vi "RT_AInoiseMeas.vi"() -> ()   [LabVIEW 2020]
uses:
  <vilib>/NI/STM/SubVIs/MetaDataElement.ctl
  <vilib>/Platform/TimedLoop/XDataNode/timing_clust.ctl
  <vilib>/Platform/TimedLoop/XDataNode/nitl_modes.ctl
  <vilib>/Platform/TimedLoop/XDataNode/wakeup.ctl
  <vilib>/NI/STM/TCP/Write Meta Data (TCP Ref).vi
  <vilib>/NI/STM/TCP/Get Connection Reference (TCP).vi
  <vilib>/NI/STM/TCP/Write Meta Data (TCP Clst).vi
  <vilib>/FPGAPlugInAG/cRIO-9064/niLvFpga_Open_cRIO-9064.vi
  <vilib>/rvi/interface/common/dynamic/niFpgaDynamicAddResources.vi
  <vilib>/NI/STM/TCP/Write Message (TCP).vi
  <vilib>/Utility/error.llb/Error Cluster From Error Code.vi
  <vilib>/rvi/errors/niLvFpgaAdjustHostInterfaceError.vi
  <vilib>/FPGAPlugInAG/Dynamic/niLvFpga_Close_Dynamic.vi
  <vilib>/rvi/interface/nirviOpenFPGA/nirviOpenFPGA.xnode
  FPGA Bitfiles/pumpmeasurements_FPGATarget2_FPGAmain_llEPu4umcUg.lvbitx
  <vilib>/rvi/interface/nirviReadWriteControl/nirviReadWriteControl.xnode
  <vilib>/Platform/TimedLoop/XDataNode/XDataNode.xnode
  <vilib>/rvi/interface/nirviCloseFPGA/nirviCloseFPGA.xnode
  <vilib>/Platform/TimedLoop/XDataNode/XDNodeRunTimeDep.lvlib
  Components_global/Timing/Timing.lvlib
  <vilib>/NI/STM/NI STM.lvlib
  <vilib>/rvi/interface/Simulation/niFpgaSimulationCallBeginRW.vi
  NiFpgaLv.dll
panel:
  out "NI9208 AI \nloop time [ms]":u32
  out "NI9205 AI \nloop time [ms]":dbl
  in  "Select channel":T1(ring)
  in  "Select Module":enum16{"NI9205", "NI9208"}(ring)
  out "RT Loop Rate":dbl format="%.3p"
  out "# of iterations\n[STM write]":i32
  out "# elements \nFIFO buffer":u32
  out "Finished \nlate counter?":dbl
  in  "stop":bool
  # "- Open PC_AINoiseMeas.vi and run that VI \nas well to start capturing data!"
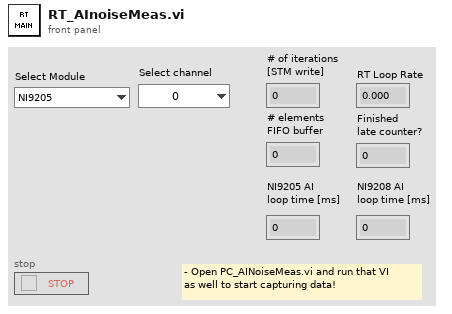
[diagram p1: front panel]
types:
  T1 = enum16{"0", "1", "2", "3", "4", "5", "6", "7", "8", "9", "10", "11", "12", "13", "14", "15"}
  T2 = typedef "NI STM.lvlib/MetaDataElement.ctl" = string
  T3 = typedef "NI STM.lvlib/TCP Connection Info.ctl" = cluster{"connection ID":refnum<k5>, "meta data":T2[]}
  T4 = typedef "XDNodeRunTimeDep.lvlib/timing_clust.ctl" = cluster{"Expected End [f-1]":u64, "Actual End [f-1]":u64, "Finished Late? [f-1]":bool, "Expected End [i-1]":u64, "Actual End [i-1]":u64, "Finished Late? [i-1]":bool, "Expected Start [i]":u64, "Actual Start [i]":u64, "Expected Start [f]":u64, "Actual Start [f]":u64, "Source Name":string, "Structure Name":string, "Period":i64, "Deadline":i64, "Offset":i64, "Start":i64, "Priority":i32, "Timeout":i32, "Mode":T5, "Wakeup Reason":T6, "Error":errorcluster, "Source Type":string, "Secondary Source Type":string, "Global End Time":u64, "Global Start Time":u64, "Frame Duration":u64, "Iteration Duration":u64, "Assigned CPU":i32, "I/O Scan Engine Mode":u32}
  T5 = typedef "XDNodeRunTimeDep.lvlib/nitl_modes.ctl" = enum32{"No Change", "Process missed periods, maintain original phase", "Discard missed periods, maintain original phase", "Process missed periods, ignore original phase", "Discard missed periods, ignore original phase"}
  T6 = typedef "XDNodeRunTimeDep.lvlib/wakeup.ctl" = enum32{"Normal", "Aborted", "Asynchronous wakeup", "Timing source error", "Timed loop error", "Timeout"}
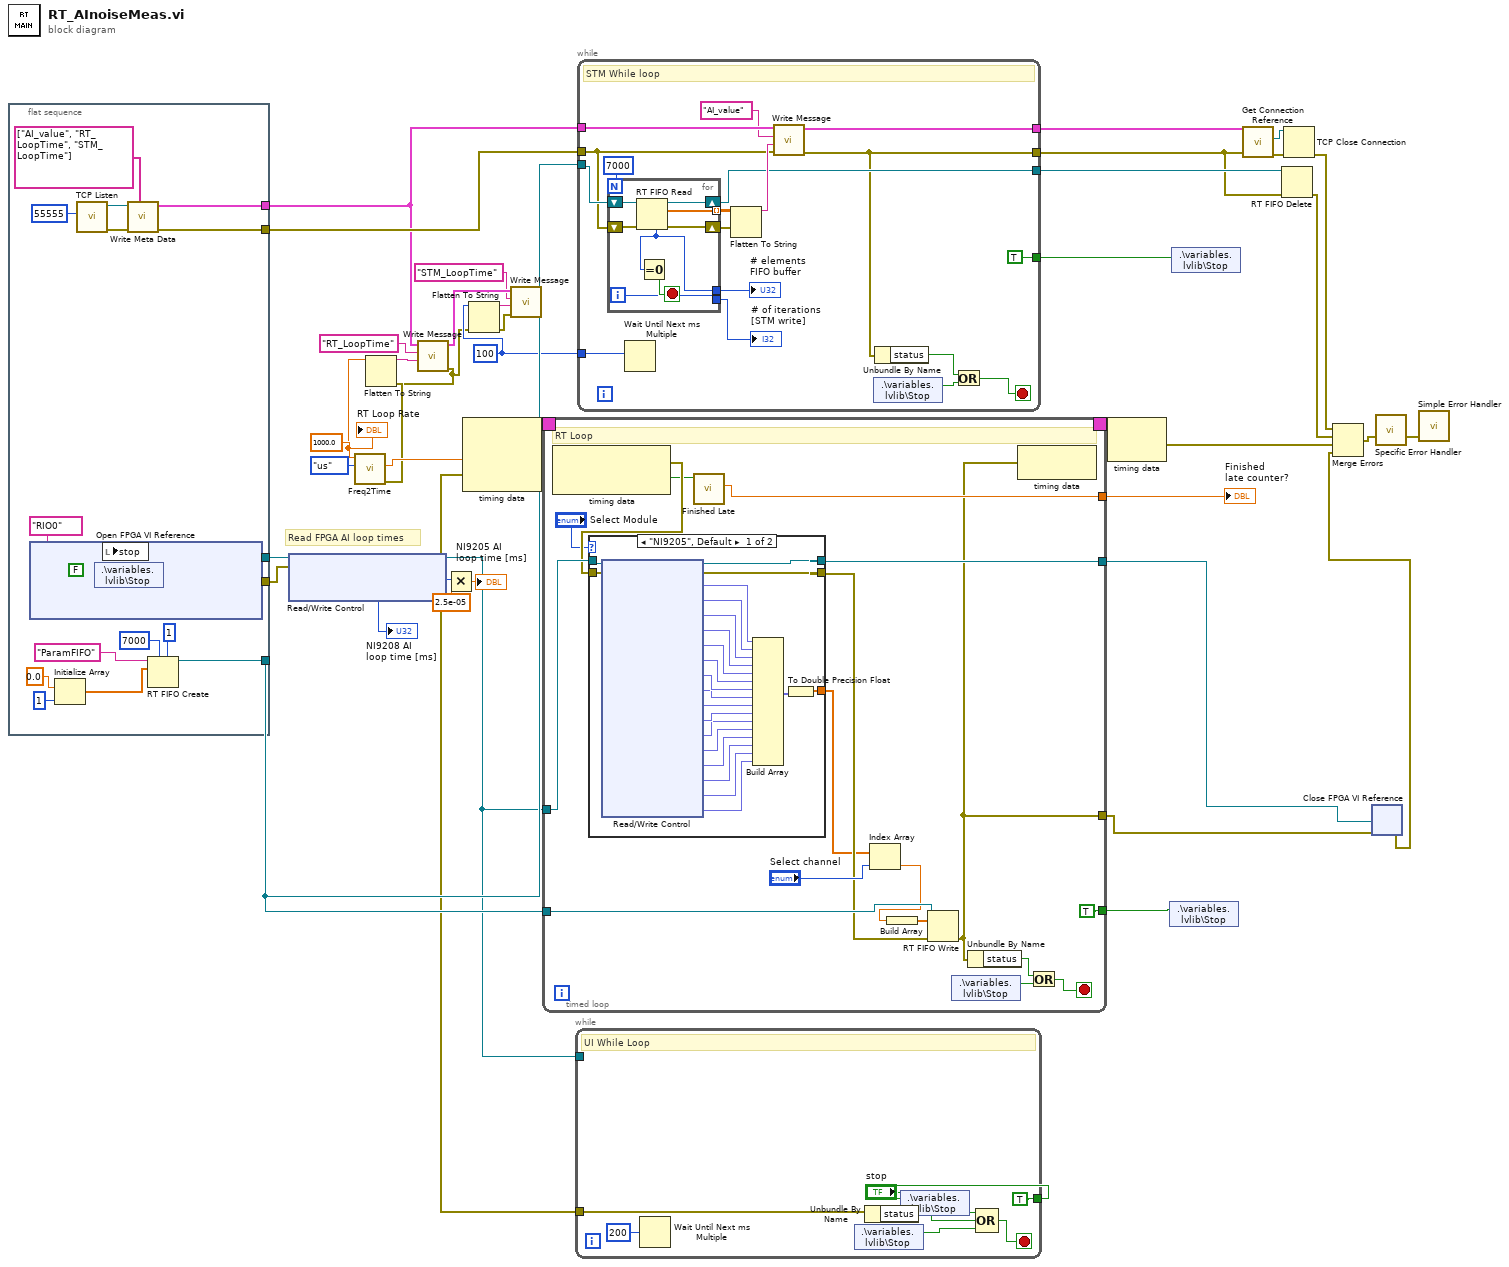
[diagram p0: block diagram]
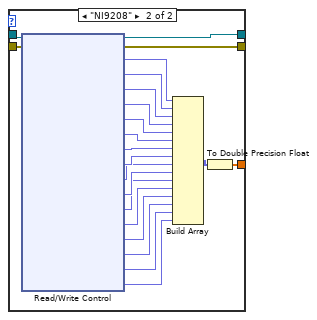
[diagram p2: hidden frame]
diagram:
  w17 = u32 100 ("millisecond multiple")
  # "Read FPGA AI loop times"
  n1 = flat-sequence {
    tunnel: [w59] -> w8
    tunnel: [w58] -> w1
    tunnel: [w53] -> w14
    tunnel: [w52] -> w37
    tunnel: [w51] -> w18
    frame #0 {
      w60 = FALSE ("Stop")
      n2 = xnode "Open FPGA VI Reference"("resource name"=tag "RIO0") -> ("FPGA VI Reference Out"=w58:refnum<k20>, "error out"=w61:errorcluster)  [unwired: 1 in]
      n3 = Initialize Array(0.0 ("element"), 1 ("dimension size")) -> (w46:dbl[])
      n4 = call <vilib>:"TCP Listen.vi"("port"=u16 55555) -> ("error out"=w56:errorcluster, "connection ID"=w55:refnum<k5>)  [unwired: 6 in, 3 out]
      n5 = shared-variable ".\\variables.lvlib\\Stop"(w60, error in=w61) -> (error out=w59:errorcluster)
      n6 = local write "stop"(w60) -> ()
      n7 = call-poly <vilib>:"Write Meta Data.vi"("meta data"=T2[] ["AI_value", "RT_LoopTime", "STM_LoopTime"], "error in"=w56, "connection ID"=w55) -> ("error out"=w52:errorcluster, "connection info out"=w53:T3)  [unwired: 7 in]
      n8 = RT FIFO Create(0:"ParamFIFO" ("name (unnamed)"), 1:w46, 4:u32 7000 ("size (10)"), 6:u32 1 ("elements in array (1)")) -> (8:w51:refnum<k33>)  [unwired: 4 in, 2 out]
    }
  }
  n9 = xnode "Read/Write Control"("FPGA VI Reference In"=w1, "error in"=w8) -> ("FPGA VI Reference Out"=w6:refnum<k20>, "error out"=w7:errorcluster, "NI9205 AI loop time [ticks]"=w2:u32, "NI9208 AI loop time [ms]"=→"NI9208 AI \nloop time [ms]":u32)
  n10 = call "Freq2Time.vi"("Int. Time Unit"=enum16{"sec", "us", "ms"}."us", "Sample rate (Hz)"=1000.0 ("Period")) -> ("error out"=w26:errorcluster, "Int.  time [unit]"=w38:dbl, "New Sample rate (Hz)"=w28:dbl)  [unwired: 7 in]
  "RT Loop Rate" <- w28
  n11 = Flatten To String(anything=w28, error in (no error)=w26) -> (data string=w29:string, error out=w16:errorcluster)  [unwired: 2 in, 1 out]
  n12 = call-poly <vilib>:"Write Message.vi"("error in"=w16, "data"=w29, "name"="RT_LoopTime", "connection info in"=w14) -> ("connection info out"=w13:T3)  [unwired: 6 in, 1 out]
  n13 = Multiply(x=w2, y=2.5e-05 ("NI9205 AI loop time [ms]")) -> (x*y=→"NI9205 AI \nloop time [ms]":dbl)
  n14 = node-c288(w38, w7) -> (w43:T4)  [unwired: 1 in]
  n15 = Flatten To String(anything=w17, error in (no error)=w16) -> (data string=w11:string, error out=w15:errorcluster)  [unwired: 2 in, 1 out]
  n16 = call-poly <vilib>:"Write Message.vi"("error in"=w15, "data"=w11, "name"="STM_LoopTime", "connection info in"=w13) -> ()  [unwired: 6 in, 2 out]
  n17 = timed-loop {
    tunnel: w6 -> [w78]
    timing: w43 -> [_]
    timing-out: [_] -> w42
    tunnel: [w75] -> w41
    tunnel: w18 -> [w74]
    tunnel: [TRUE ("Stop")] -> w20
    tunnel: [w66] -> w10
    tunnel: [w65] -> w9
    stop <- w72 stop-if-true
    # "RT Loop"
    n18 = node-c288() -> (w77:errorcluster, w76:bool)  [unwired: 1 in]
    n19 = case shown="\"NI9205\", Default" "Select Module" {
      tunnel: w78 -> [w100 w122]
      tunnel: w77 -> [w99 w120]
      tunnel: [w79 w103] -> w63
      tunnel: [w98 w121] -> w66
      tunnel: [w97 w119] -> w68
      frame "NI9205", Default {
        n20 = xnode "Read/Write Control"("FPGA VI Reference In"=w100, "error in"=w99) -> ("FPGA VI Reference Out"=w98:refnum<k20>, "error out"=w97:errorcluster, "NI9205: AI0 [V]"=w96:fxp<+/-,35,5>, "NI9205: AI1 [V]"=w95:fxp<+/-,35,5>, "NI9205: AI2 [V]"=w94:fxp<+/-,35,5>, "NI9205: AI3 [V]"=w93:fxp<+/-,35,5>, "NI9205: AI4 [V]"=w92:fxp<+/-,35,5>, "NI9205: AI5 [V]"=w91:fxp<+/-,35,5>, "NI9205: AI6 [V]"=w90:fxp<+/-,35,5>, "NI9205: AI7 [V]"=w89:fxp<+/-,35,5>, "NI9205: AI16 [V]"=w88:fxp<+/-,35,5>, "NI9205: AI17 [V]"=w87:fxp<+/-,35,5>, "NI9205: AI18 [V]"=w86:fxp<+/-,35,5>, "NI9205: AI19 [V]"=w85:fxp<+/-,35,5>, "NI9205: AI20 [V]"=w84:fxp<+/-,35,5>, "NI9205: AI21 [V]"=w83:fxp<+/-,35,5>, "NI9205: AI22 [V]"=w82:fxp<+/-,35,5>, "NI9205: AI23 [V]"=w81:fxp<+/-,35,5>)
        n21 = Build Array(w96, w95, w94, w93, w92, w91, w90, w89, w88, w87, w86, w85, w84, w83, w82, w81) -> (w80:fxp<+/-,35,5>[])
        n22 = To Double Precision Float(number=w80) -> (double precision float=w79:dbl[])
      }
      frame "NI9208" {
        n23 = xnode "Read/Write Control"("FPGA VI Reference In"=w122, "error in"=w120) -> ("FPGA VI Reference Out"=w121:refnum<k20>, "error out"=w119:errorcluster, "NI9208: AI0 [A]"=w101:fxp<+/-,24,-4>, "NI9208: AI1 [A]"=w118:fxp<+/-,24,-4>, "NI9208: AI2 [A]"=w117:fxp<+/-,24,-4>, "NI9208: AI3 [A]"=w116:fxp<+/-,24,-4>, "NI9208: AI4 [A]"=w115:fxp<+/-,24,-4>, "NI9208: AI5 [A]"=w114:fxp<+/-,24,-4>, "NI9208: AI6 [A]"=w113:fxp<+/-,24,-4>, "NI9208: AI7 [A]"=w112:fxp<+/-,24,-4>, "NI9208: AI8 [A]"=w111:fxp<+/-,24,-4>, "NI9208: AI9 [A]"=w110:fxp<+/-,24,-4>, "NI9208: AI10 [A]"=w109:fxp<+/-,24,-4>, "NI9208: AI11 [A]"=w108:fxp<+/-,24,-4>, "NI9208: AI12 [A]"=w107:fxp<+/-,24,-4>, "NI9208: AI13 [A]"=w106:fxp<+/-,24,-4>, "NI9208: AI14 [A]"=w105:fxp<+/-,24,-4>, "NI9208: AI15 [A]"=w104:fxp<+/-,24,-4>)
        n24 = Build Array(w101, w118, w117, w116, w115, w114, w113, w112, w111, w110, w109, w108, w107, w106, w105, w104) -> (w102:fxp<+/-,24,-4>[])
        n25 = To Double Precision Float(number=w102) -> (double precision float=w103:dbl[])
      }
    }
    n26 = call "Finished Late.vi"("Finished \nLate?"=w76) -> ("# Finished\nLate counter"=w75:dbl)  [unwired: 8 in, 2 out]
    n27 = Index Array(array=w63, index="Select channel") -> (element=w64:dbl)
    n28 = Build Array(w64) -> (w62:dbl[])
    n29 = RT FIFO Write(0:w74, 1:w62, 3:w68) -> (11:w65:errorcluster)  [unwired: 2 in, 3 out]
    n30 = shared-variable ".\\variables.lvlib\\Stop"() -> (w71:bool)  [unwired: 1 in, 1 out]
    n31 = Unbundle By Name(w65) -> ("status"=w70:bool)
    n32 = node-c288(w65) -> ()  [unwired: 1 out]
    n33 = Or(x=w70, y=w71) -> (x .or. y?=w72:bool)
  }
  "Finished \nlate counter?" <- w41
  n34 = while {
    tunnel: w7 -> [w131]
    tunnel: w6 -> [_]
    tunnel: [TRUE ("Stop")] -> w19
    stop <- w132 stop-if-true
    # "UI While Loop"
    n35 = Wait Until Next ms Multiple(millisecond multiple=u32 200) -> ()  [unwired: 1 out]
    n36 = shared-variable ".\\variables.lvlib\\Stop"() -> (w133:bool)  [unwired: 1 in, 1 out]
    n37 = Unbundle By Name(w131) -> ("status"=w130:bool)
    n38 = Compound Arithmetic op=OR("stop", w130, w133) -> (w132:bool)
  }
  n39 = while {
    tunnel: w14 -> [w153]
    tunnel: w37 -> [w147]
    tunnel: [w151] -> w36
    tunnel: [w137] -> w32
    tunnel: w18 -> [w149]
    tunnel: [w146] -> w33
    tunnel: [TRUE ("Stop")] -> w21
    tunnel: w17 -> [w136]
    stop <- w139 stop-if-true
    # "STM While loop"
    n40 = for {
      N: 7000 -> [_]
      shift-right: [w158] -> w146
      shift-left: w149 -> [w161]
      shift-right: [w160] -> w148
      shift-left: w147 -> [w159]
      tunnel: [w157] -> w145
      tunnel: [w155] -> w144
      tunnel: [w154] -> w143 mode=indexing
      i -> [w155]
      stop <- w156 stop-if-true
      n41 = RT FIFO Read(0:w161, 3:w159) -> (7:w157:u32, 8:w158:refnum<k33>, 9:w154:dbl[], 11:w160:errorcluster)  [unwired: 2 in, 1 out]
      n42 = Equal To 0?(x=w157) -> (x = 0?=w156:bool)
    }
    "# elements \nFIFO buffer" <- w145
    "# of iterations\n[STM write]" <- w144
    n43 = Wait Until Next ms Multiple(millisecond multiple=w136) -> ()  [unwired: 1 out]
    n44 = Flatten To String(anything=w143, error in (no error)=w148) -> (data string=w150:string)  [unwired: 2 in, 2 out]
    n45 = call-poly <vilib>:"Write Message.vi"("error in"=w147, "data"=w150, "name"="AI_value", "connection info in"=w153) -> ("error out"=w137:errorcluster, "connection info out"=w151:T3)  [unwired: 6 in]
    n46 = shared-variable ".\\variables.lvlib\\Stop"() -> (w140:bool)  [unwired: 1 in, 1 out]
    n47 = Unbundle By Name(w137) -> ("status"=w138:bool)
    n48 = Or(x=w138, y=w140) -> (x .or. y?=w139:bool)
  }
  n49 = shared-variable ".\\variables.lvlib\\Stop"(w19) -> ()  [unwired: 1 in, 1 out]
  n50 = node-c288(w42) -> (w27:errorcluster)
  n51 = shared-variable ".\\variables.lvlib\\Stop"(w20) -> ()  [unwired: 1 in, 1 out]
  n52 = shared-variable ".\\variables.lvlib\\Stop"(w21) -> ()  [unwired: 1 in, 1 out]
  n53 = call-poly <vilib>:"Get Connection Reference.vi"("error in"=w32, "connection info in"=w36) -> ("error out"=w35:errorcluster, "connection ID out"=w34:refnum<k5>)  [unwired: 7 in, 1 out]
  n54 = RT FIFO Delete(0:w33, 3:w32) -> (11:w31:errorcluster)  [unwired: 1 in]
  n55 = TCP Close Connection(connection ID=w34, error in (no error)=w35) -> (error out=w23:errorcluster)  [unwired: 1 in, 1 out]
  n56 = xnode "Close FPGA VI Reference"("FPGA VI Reference In"=w10, "error in"=w9) -> ("error out"=w22:errorcluster)
  n57 = Merge Errors(w23, w31, w27, w22) -> (w25:errorcluster)
  n58 = call "Specific Error Handler"("Error to Check"=w25) -> ("error out"=w24:errorcluster)  [unwired: 11 in, 3 out]
  n59 = call <vilib>:"Simple Error Handler.vi"("error in (no error)"=w24) -> ()  [unwired: 4 in, 5 out]
